vi "ramp.vi"(10 "reset":bool, 11 "Coagulant":T1={"flocculator volume (L)"=100.0, "clarifier volume (L)"=0.0, "dose updates per HRT"=0, "target clarified turbidity (NTU)"=0.3, "Coagulant mode"=enum."manual", "Coag dose [mg/L]"=0.0, "pump mL/rev"=0.0, "clarifier flow [L/s]"=0.5, "min Coag dose [mg/L]"=0.0, "max Coag dose [mg/L]"=0.0, "Steps"=3, "HRT response delay"=1, "Ku*"=1.0, "DOM coag demand [mg/L]"=0.0, "min DOM coag demand [mg/L]"=0.0, "max DOM coag demand [mg/L]"=0.0} {"max DOM coag demand [mg/L]" min=0.0 max=20.0 step=0.1; "min DOM coag demand [mg/L]" min=0.0 max=10.0 step=0.1; "DOM coag demand [mg/L]" min=0.0 max=20.0 step=0.1; "HRT response delay" min=1 max=10 step=1; "Steps" min=3 step=1; "clarifier flow [L/s]" min=0.0001 max=1.0 step=0.0001; "target clarified turbidity (NTU)" min=0.1 max=5.0 step=0.01; "dose updates per HRT" min=1 max=100 step=1}) -> (3 "Coag dose":dbl)   [LabVIEW 2019]
uses:
  coag.ctl
  model type.ctl
panel:
  out "Numeric":i64
  # "ramp controls"
  # "min"
  # "max"
  # "min"
  # "max"
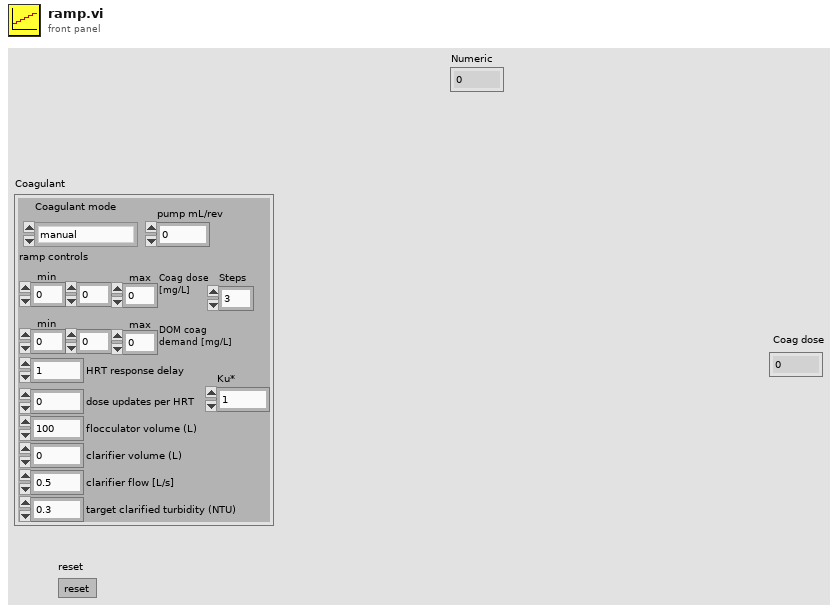
[diagram p1: front panel]
types:
  T1 = typedef "coag.ctl" = cluster{"flocculator volume (L)":dbl, "clarifier volume (L)":dbl, "dose updates per HRT":u16, "target clarified turbidity (NTU)":dbl, "Coagulant mode":T2, "Coag dose [mg/L]":dbl, "pump mL/rev":dbl, "clarifier flow [L/s]":dbl, "min Coag dose [mg/L]":dbl, "max Coag dose [mg/L]":dbl, "Steps":u16, "HRT response delay":u32, "Ku*":dbl, "DOM coag demand [mg/L]":dbl, "min DOM coag demand [mg/L]":dbl, "max DOM coag demand [mg/L]":dbl}
  T2 = typedef "model type.ctl" = enum16{"manual", "ramp", "simple corrector"}
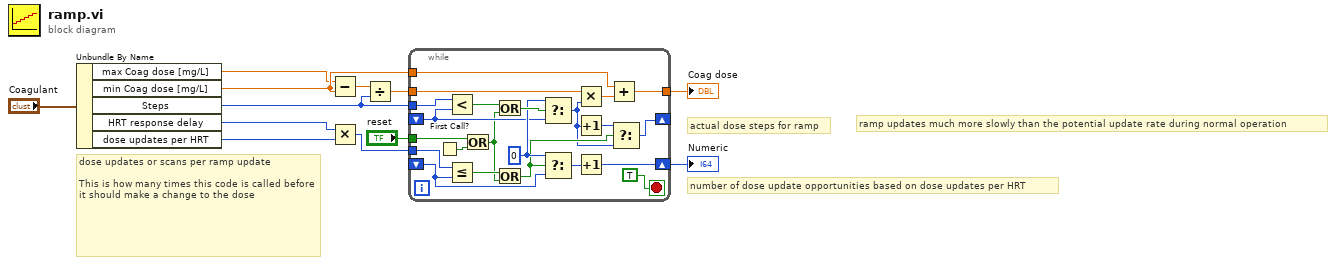
[diagram p0: block diagram]
diagram:
  # "ramp updates much more slowly than the potential update rate during normal operation"
  # "actual dose steps for ramp"
  # "number of dose update opportunities based on dose updates per HRT"
  # "dose updates or scans per ramp update\n\nThis is how many times this code is called before it should make a change to the dose"
  n1 = Unbundle By Name("Coagulant") -> ("max Coag dose [mg/L]"=w8:dbl, "min Coag dose [mg/L]"=w11:dbl, "Steps"=w2:u16, "HRT response delay"=w6:u32, "dose updates per HRT"=w5:u16)
  n2 = Subtract(x=w8, y=w11) -> (x-y=w10:dbl)
  n3 = Multiply(x=w6, y=w5) -> (x*y=w4:u32)
  n4 = Divide(x=w10, y=w2) -> (x/y=w9:dbl)
  n5 = while {
    tunnel: w11 -> [w29]
    tunnel: w9 -> [w31]
    shift-right: [w17] -> _
    shift-left: _ -> [w19]
    tunnel: w4 -> [w33]
    tunnel: [w28] -> w7
    shift-right: [w26] -> w3
    shift-left: _ -> [w25]
    tunnel: w2 -> [w24]
    tunnel: "reset" -> [w13]
    stop <- TRUE stop-if-true
    w20 = i64 0 ("t")
    n6 = First Call?() -> (First Call?: T/F=w22:bool)
    n7 = Less?(x=w24, y=w19) -> (x < y?=w23:bool)
    n8 = Less Or Equal?(x=w33, y=w25) -> (x <= y?=w32:bool)
    n9 = Or(x=w13, y=w22) -> (x .or. y?=w14:bool)
    n10 = Or(x=w23, y=w14) -> (x .or. y?=w21:bool)
    n11 = Or(x=w32, y=w14) -> (x .or. y?=w16:bool)
    n12 = Select(t=w20, s=w21, f=w19) -> (s? t:f=w15:i64)
    n13 = Select(t=w20, s=w16, f=w25) -> (s? t:f=w27:i64)
    n14 = Multiply(x=w31, y=w15) -> (x*y=w30:dbl)
    n15 = Increment(x=w15) -> (x+1=w18:i64)
    n16 = Increment(x=w27) -> (x+1=w26:i64)
    n17 = Add(x=w29, y=w30) -> (x+y=w28:dbl)
    n18 = Select(t=w18, s=w16, f=w15) -> (s? t:f=w17:i64)
  }
  "Coag dose" <- w7
  "Numeric" <- w3
